vi "Is Finite.vi"(1 "Numeric":dbl) -> (0 "is finite?":bool)   [LabVIEW 2020]
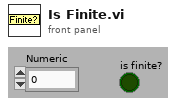
[diagram p1: front panel]
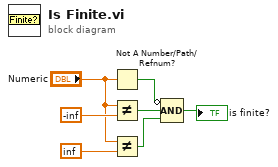
[diagram p0: block diagram]
diagram:
  n1 = Not A Number/Path/Refnum?(number/path/refnum="Numeric") -> (NaN/Path/Refnum?=w1:bool)
  n2 = Not Equal?(x="Numeric", y=-inf) -> (x != y?=w5:bool)
  n3 = Not Equal?(x="Numeric", y=inf) -> (x != y?=w4:bool)
  n4 = Compound Arithmetic op=AND(invert w1, w5, w4) -> (→"is finite?":bool)
